vi "42 Confing File Read GPS Time (x64-2018).vi"() -> (4 "GPS Time":string, 6 "GPS Date":string, 8 "Labview Time":dbl format="%.2f", 10 "CPU Time":dbl format="%.2f", 14 "GPS Lock":bool, 15 "Tick Count":dbl format="%.2f")   [LabVIEW 2017]
uses:
  <vilib>/Utility/config.llb/Read Key (Double).vi
  <vilib>/Utility/config.llb/Read Key (String).vi
  <vilib>/Utility/config.llb/Read Key (Boolean).vi
  <vilib>/Utility/config.llb/NI_LVConfig.lvlib
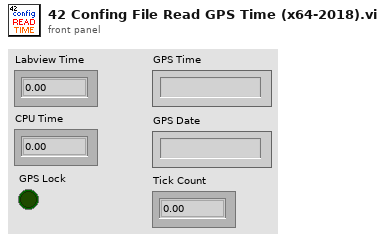
[diagram p1: front panel]
types:
  T1 = typedef "NI_LVConfig.lvlib/Config Data RefNum.ctl" = refnum<k1>
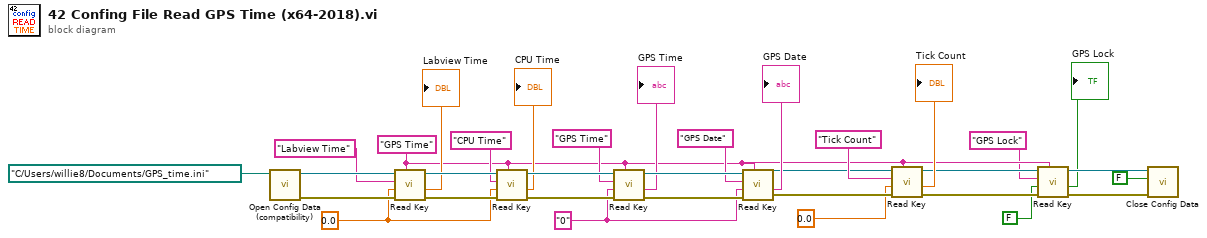
[diagram p0: block diagram]
diagram:
  w20 = "0" ("key")
  w21 = 0.0
  w8 = "GPS Time" ("section")
  n1 = call <vilib>:"Open Config Data (compatibility).vi"("configuration file path"=path "C:/Users/willie8/Documents/GPS_time.ini") -> ("error out"=w32:errorcluster, "refnum"=w33:T1)  [unwired: 8 in, 1 out]
  n2 = call-poly <vilib>:"Read Key.vi"("section"=w8, "error in (no error)"=w32, "default value"=w21, "key"="Labview Time", "refnum"=w33) -> ("error out"=w28:errorcluster, "value"=→"Labview Time":dbl, "refnum out"=w30:T1)  [unwired: 3 in, 1 out]
  n3 = call-poly <vilib>:"Read Key.vi"("section"=w8, "error in (no error)"=w28, "default value"=w21, "key"="CPU Time", "refnum"=w30) -> ("error out"=w26:errorcluster, "value"=→"CPU Time":dbl, "refnum out"=w27:T1)  [unwired: 3 in, 1 out]
  n4 = call-poly <vilib>:"Read Key.vi"("section"=w8, "error in (no error)"=w26, "default value"=w20, "key"="GPS Time", "refnum"=w27) -> ("error out"=w23:errorcluster, "value"=→"GPS Time":string, "refnum out"=w24:T1)  [unwired: 3 in, 1 out]
  n5 = call-poly <vilib>:"Read Key.vi"("section"=w8, "error in (no error)"=w23, "default value"=w20, "key"="GPS Date", "refnum"=w24) -> ("error out"=w13:errorcluster, "value"=→"GPS Date":string, "refnum out"=w14:T1)  [unwired: 3 in, 1 out]
  n6 = call-poly <vilib>:"Read Key.vi"("section"=w8, "error in (no error)"=w13, "default value"=0.0, "key"="Tick Count", "refnum"=w14) -> ("error out"=w7:errorcluster, "value"=→"Tick Count":dbl, "refnum out"=w9:T1)  [unwired: 3 in, 1 out]
  n7 = call-poly <vilib>:"Read Key.vi"("section"=w8, "error in (no error)"=w7, "default value"=FALSE, "key"="GPS Lock", "refnum"=w9) -> ("error out"=w6:errorcluster, "value"=→"GPS Lock":bool, "refnum out"=w5:T1)  [unwired: 3 in, 1 out]
  n8 = call <vilib>:"Close Config Data.vi"("error in (no error)"=w6, "write file if changed (T)"=FALSE ("write configuration file? (T)"), "refnum"=w5) -> ()  [unwired: 7 in, 2 out]
